vi "Get_Power_Measurement_Utility.vi"() -> ()   [LabVIEW 2015]
panel:
  out "Measurement":dbl
  in  "Cal Route":string[](array[string])=["SP_PWR_SENSOR_to_TX1"]
  in  "Rnd?":bool
  in  "Frequency":dbl=1000000000.0
  in  "Cal?":bool=TRUE
  out "error out":errorcluster
  in  "VISA Refnum in":refnum<visa-resource-name>="PwrSensor_1"
  in  "error in (no error)":errorcluster
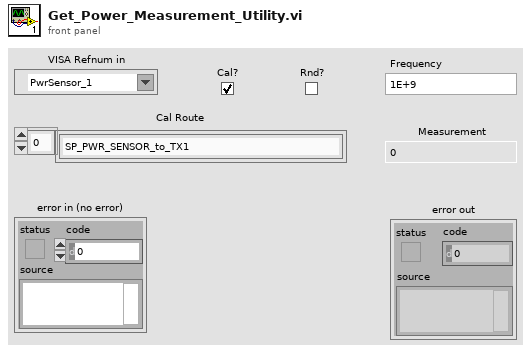
[diagram p1: front panel]
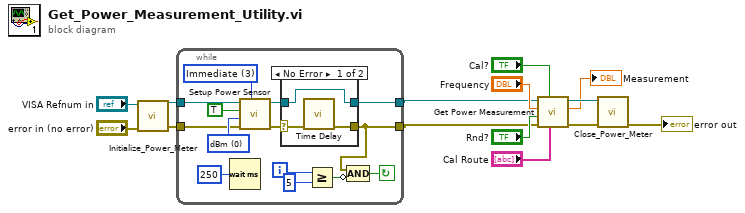
[diagram p0: block diagram]
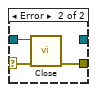
[diagram p2: hidden frame]
diagram:
  n1 = call "Initialize_Power_Meter.vi"("error in (no error)"="error in (no error)", "VISA Refnum in"="VISA Refnum in") -> ("error out"=w3:errorcluster, "VISA resource name out"=w4:refnum<visa-resource-name>)  [unwired: 8 in]
  n2 = while {
    tunnel: [w21] -> w1
    tunnel: [w28] -> w2
    tunnel: w4 -> [w16]
    tunnel: w3 -> [w15]
    i -> [w24]
    stop <- w20 continue-if-true
    w19 = 3 items=["Bus", "External", "Hold", "Immediate", "Internal A"] ("Trigger Source")
    w18 = u16 0 items=["dBm", "W"] ("Units")
    n3 = Wait (ms)(milliseconds to wait=u32 250) -> ()  [unwired: 1 out]
    n4 = call "Setup Power Sensor.vi"("Trigger Source"=w19, "error in (no error)"=w15, "Units"=w18, "Enable Initiate Continuous"=TRUE, "VISA Refnum in"=w16) -> ("error out"=w25:errorcluster, "VISA Refnum out"=w26:refnum<visa-resource-name>)  [unwired: 5 in]
    n5 = case shown="No Error" w25 {
      selector: w25 -> [w31 w32]
      tunnel: [w30 w34] -> w21
      tunnel: w26 -> [w29 w33]
      tunnel: [w29 _] -> w28
      frame No Error {
        n6 = call "Time Delay"("error in (no error)"=w31) -> ("error out"=w30:errorcluster)  [unwired: 10 in]
      }
      frame Error {
        n7 = call <instrlib>:"Close.vi"("error in (no error)"=w32, "VISA resource name"=w33) -> ("error out"=w34:errorcluster)  [unwired: 9 in]
      }
    }
    n8 = Greater Or Equal?(x=w24, y=5) -> (x >= y?=w22:bool)
    n9 = Compound Arithmetic op=AND(w21, invert w22) -> (w20:bool)
  }
  n10 = call "Get Power Measurement.vi"("Cal Route"="Cal Route", "Cal?"="Cal?", "error in (no error)"=w1, "Rnd?"="Rnd?", "Frequency"="Frequency", "VISA Refnum in"=w2) -> ("error out"=w12:errorcluster, "Measurement"=→"Measurement":dbl, "VISA Refnum out"=w11:refnum<visa-resource-name>)  [unwired: 3 in]
  n11 = call "Close_Power_Meter.vi"("error in (no error)"=w12, "VISA resource name"=w11) -> ("error out"=→"error out":errorcluster)  [unwired: 9 in]
